vi "CFTS-Options Dialog.vi"(0 "Options in":T1, 2 "Parent VI":refnum<vi>) -> (4 "Options out":T1, 10 "Cancelled?":bool=TRUE)   [LabVIEW 2020]
doc: "Use this template to create a dialog box with event handling."
uses:
  epl-vi-lib/Utility VIs/Controls/KBackground Gradient/KBackground Gradient.xctl
  CFTS-Options.ctl
  epl-vi-lib/Utility VIs/Controls/KListboxEx/KListboxEx.xctl
panel:
  in  "Root data folder":path
  in  "Allow nonEPL":bool caption="Allow non-EPL compatible"
  in  "Names":i32(xcontrol)
  in  "Allow all users":bool
  in  "Users":i32(xcontrol)
  in  "Password":bool
  in  "Extension":string caption="Default data file extension"
  in  "Rig name":string
  in  "Help Button":bool
  in  "background":dbl(xcontrol)
  in  "Vitals":bool caption="Auto-start physiological monitor"
  in  "Left":u16(ring) items=["57TTH", "TTH66"]
  in  "Right":u16(ring) items=["57TTH", "TTH66"]
  in  "Cancel":bool
  in  "OK":bool
  # "Options"
  # "Acoustic System IDs"
  # "Other options"
  # "Advanced users"
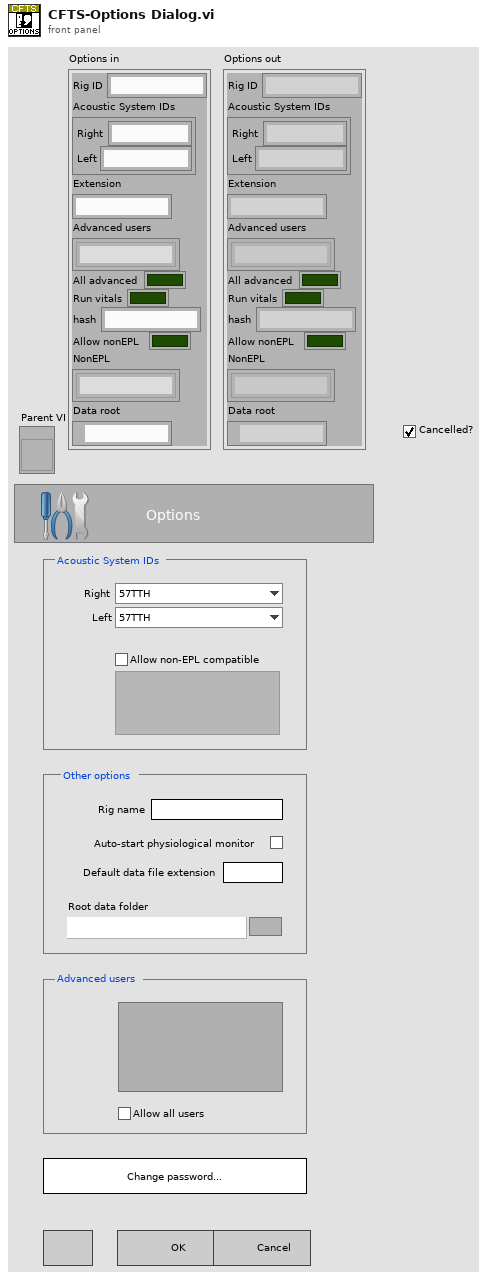
[diagram p1: front panel]
types:
  T1 = typedef "CFTS-Options.ctl" = cluster{"Rig ID":string, "Acoustic System IDs":cluster{"Right":string, "Left":string}, "Extension":string, "Advanced users":string[], "All advanced":bool, "Run vitals":bool, "hash":string, "Allow nonEPL":bool, "NonEPL":string[], "Data root":path}
  T2 = enum8{"Enabled", "Disabled", "Disabled and Grayed Out"}
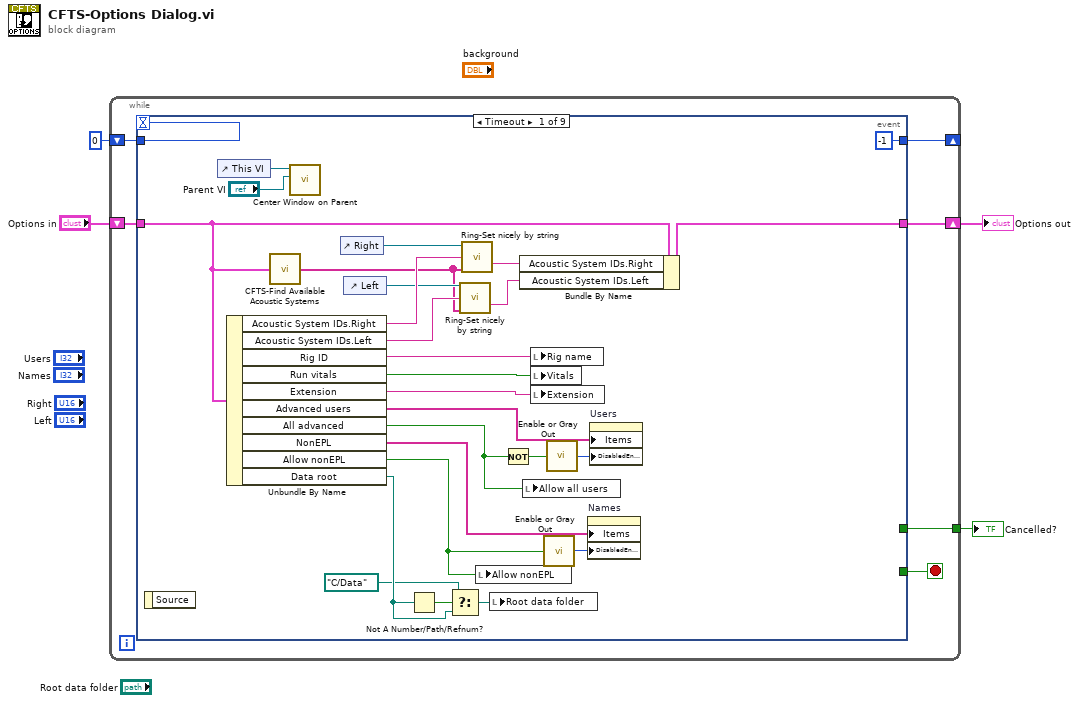
[diagram p0: block diagram]
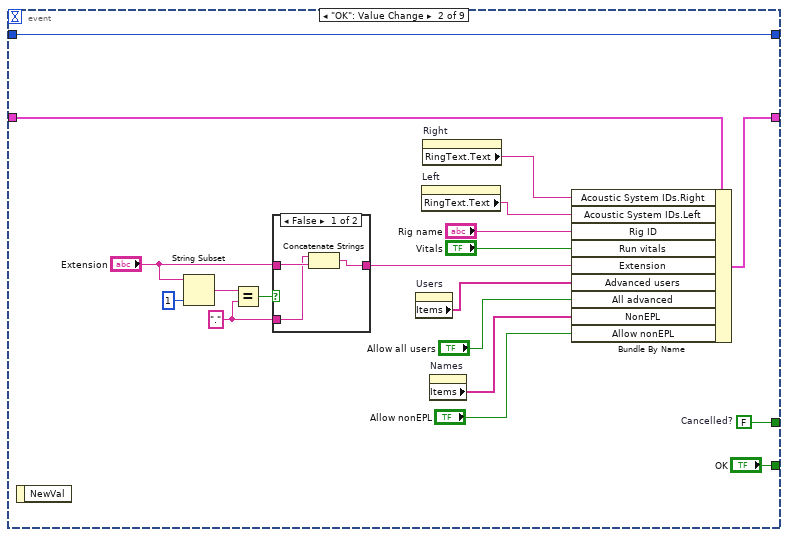
[diagram p2: hidden frame]
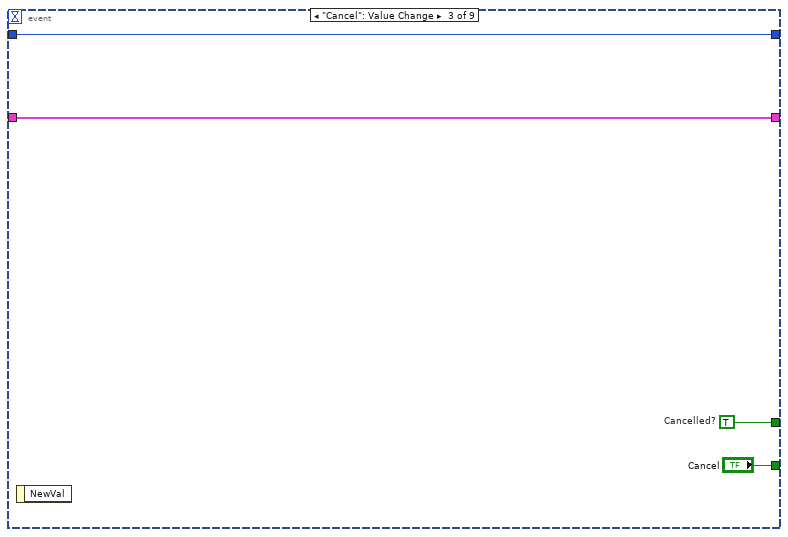
[diagram p4: hidden frame]
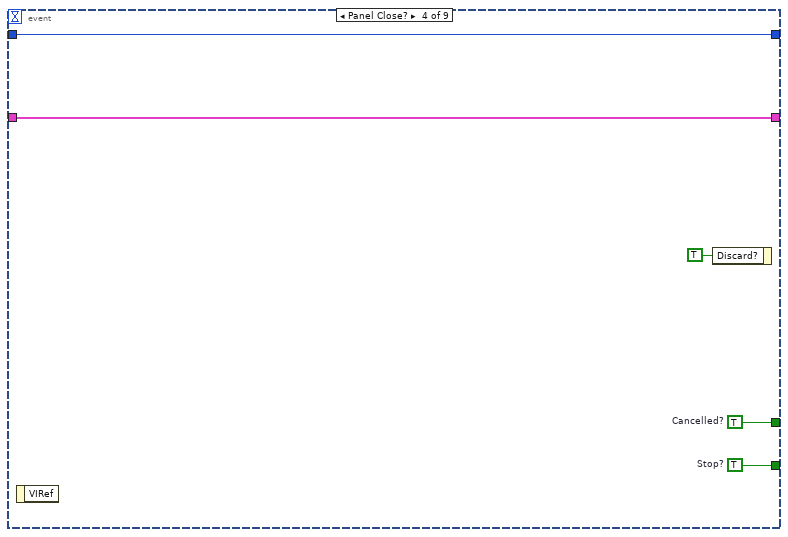
[diagram p5: hidden frame]
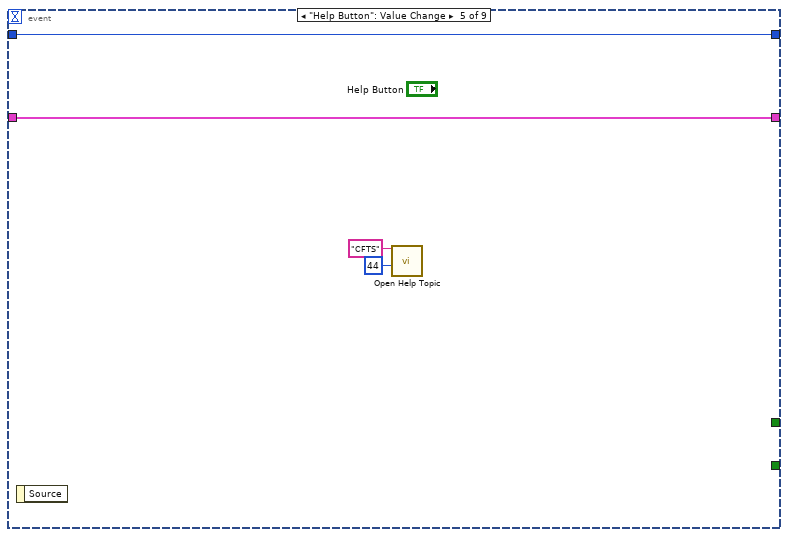
[diagram p6: hidden frame]
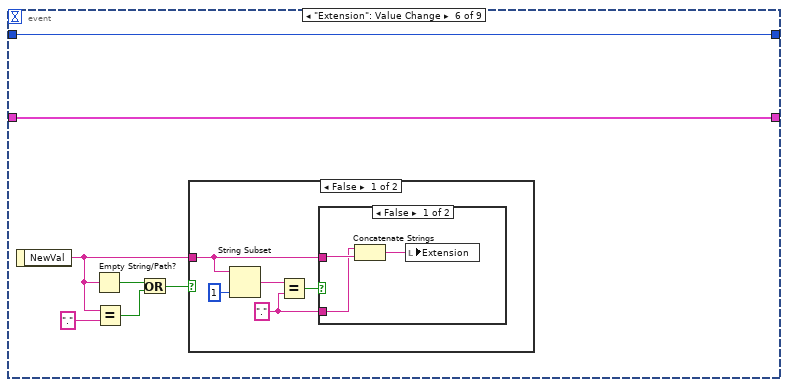
[diagram p7: hidden frame]
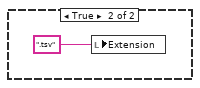
[diagram p9: hidden frame]
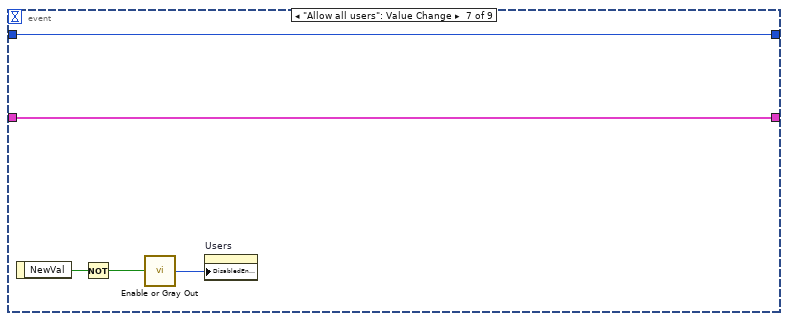
[diagram p10: hidden frame]
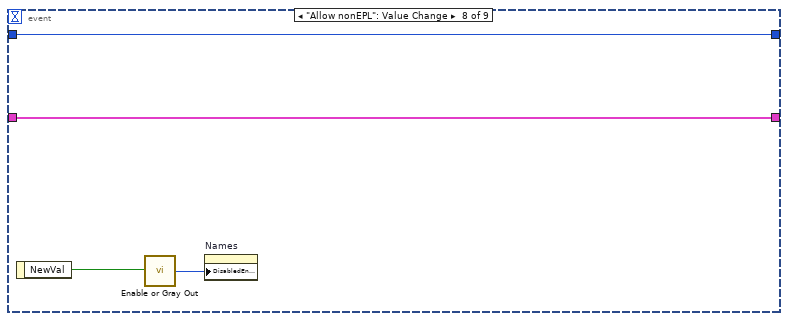
[diagram p11: hidden frame]
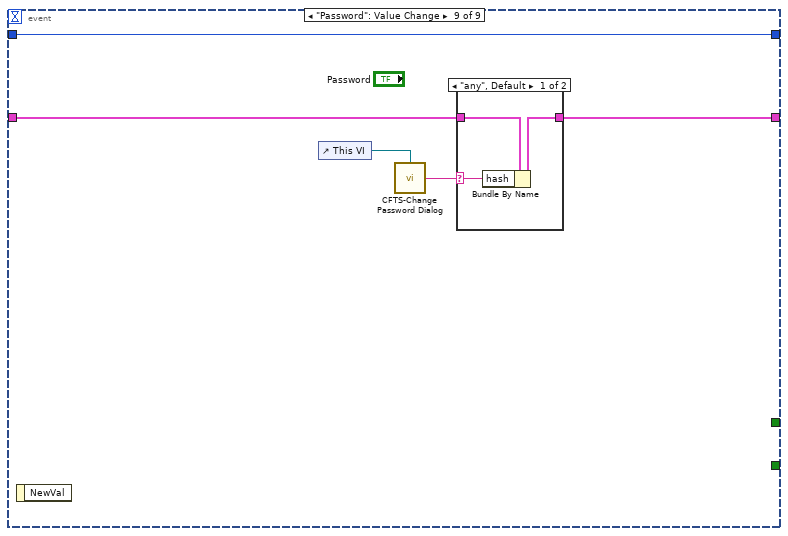
[diagram p12: hidden frame]
diagram:
  n1 = while {
    tunnel: [w9] -> w4
    shift-right: [w8] -> _
    shift-left: 0 -> [w7]
    shift-right: [w6] -> w1
    shift-left: "Options in" -> [w5]
    stop <- w10 stop-if-true
    n2 = event shown="[0] Timeout" {
      selector: _ -> [_ _ _ _ _ _ _ _ _]
      dyn-events: _ -> [_ _ _ _ _ _ _ _ _]
      timeout: w7 -> [_ _ _ _ _ _ _ _ _]
      tunnel: [_ "OK" "Cancel" w67 _ _ _ _ _] -> w10
      tunnel: [_ w55 w63 w66 _ _ _ _ _] -> w9
      tunnel: [-1 w52 w61 w65 w72 w79 w93 w97 w102] -> w8
      tunnel: w7 -> [_ w52 w61 w65 w72 w79 w93 w97 w102]
      tunnel: [w19 w45 w60 w64 w71 w78 w92 w96 w98] -> w6
      tunnel: w5 -> [w15 w51 w60 w64 w71 w78 w92 w96 w100]
      event Timeout {
        n3 = event-data() -> ()  [unwired: 1 in, 1 out]
        n4 = control-ref of="This VI"() -> (w32:refnum<vi>)
        n5 = Unbundle By Name(w15) -> ("Acoustic System IDs.Right"=w22:string, "Acoustic System IDs.Left"=w21:string, "Rig ID"=w33:string, "Run vitals"=w35:bool, "Extension"=w34:string, "Advanced users"=w30:string[], "All advanced"=w28:bool, "NonEPL"=w26:string[], "Allow nonEPL"=w24:bool, "Data root"=w12:path)
        n6 = call "CFTS-Find Available Acoustic Systems.vi"("Options"=w15) -> ("Acoustic Systems"=w16:string[])  [unwired: 14 in]
        n7 = call "Center Window on Parent.vi"("Parent VI"="Parent VI", "VI in"=w32) -> ()  [unwired: 8 in, 2 out]
        n8 = control-ref of="Right"() -> (w23:refnum<vi>)
        n9 = control-ref of="Left"() -> (w20:refnum<vi>)
        n10 = Not A Number/Path/Refnum?(number/path/refnum=w12) -> (NaN/Path/Refnum?=w14:bool)
        n11 = Select(t=path "C:/Data", s=w14, f=w12) -> (s? t:f=w13:path)
        n12 = call "Ring-Set nicely by string.vi"("Ring in"=w20, "Device"=w21, "Strings []"=w16) -> ("Selection"=w17:string)  [unwired: 8 in, 4 out]
        n13 = call "Ring-Set nicely by string.vi"("Ring in"=w23, "Device"=w22, "Strings []"=w16) -> ("Selection"=w18:string)  [unwired: 8 in, 4 out]
        n14 = local write "Allow nonEPL"(w24) -> ()
        n15 = local write "Root data folder"(w13) -> ()
        n16 = Not(x=w28) -> (.not. x?=w27:bool)
        n17 = Bundle By Name(cluster=w15, "Acoustic System IDs.Right"=w18, "Acoustic System IDs.Left"=w17) -> (w19:T1)
        n18 = local write "Allow all users"(w28) -> ()
        n19 = local write "Rig name"(w33) -> ()
        n20 = local write "Vitals"(w35) -> ()
        n21 = local write "Extension"(w34) -> ()
        n22 = call "Enable or Gray Out.vi"("Boolean"=w24) -> ("Disabled"=w25:T2)
        n23 = call "Enable or Gray Out.vi"("Boolean"=w27) -> ("Disabled"=w29:T2)
        n24 = property on="Names" class="KListboxEx (strict)"("Items"=w26, "DisabledEnum"=w25) -> ()  [unwired: 2 in, 2 out]
        n25 = property on="Users" class="KListboxEx (strict)"("Items"=w30, "DisabledEnum"=w29) -> ()  [unwired: 2 in, 2 out]
      }
      event "OK": Value Change {
        w46 = "."
        w55 = FALSE  # Cancelled?
        n26 = event-data() -> ()  [unwired: 1 in, 1 out]
        n27 = String Subset(string="Extension", length (rest)=1 ("length (rest)")) -> (substring=w49:string)  [unwired: 1 in]
        n28 = Equal?(x=w49, y=w46) -> (x = y?=w48:bool)
        n29 = case shown="False" w48 {
          tunnel: "Extension" -> [w58 w59]
          tunnel: w46 -> [w57 _]
          tunnel: [w56 w59] -> w43
          frame False {
            n30 = Concatenate Strings(w57, w58) -> (w56:string)
          }
          frame True {
          }
        }
        n31 = property on="Users" class="KListboxEx (strict)"() -> ("Items"=w42:string[])  [unwired: 2 in, 2 out]
        n32 = property on="Left" class="Ring (strict)"() -> ("RingText.Text"=w37:string)  [unwired: 2 in, 2 out]
        n33 = property on="Right" class="Ring (strict)"() -> ("RingText.Text"=w38:string)  [unwired: 2 in, 2 out]
        n34 = property on="Names" class="KListboxEx (strict)"() -> ("Items"=w40:string[])  [unwired: 2 in, 2 out]
        n35 = Bundle By Name(cluster=w51, "Acoustic System IDs.Right"=w38, "Acoustic System IDs.Left"=w37, "Rig ID"="Rig name", "Run vitals"="Vitals", "Extension"=w43, "Advanced users"=w42, "All advanced"="Allow all users", "NonEPL"=w40, "Allow nonEPL"="Allow nonEPL") -> (w45:T1)
      }
      event "Cancel": Value Change {
        w63 = TRUE  # Cancelled?
        n36 = event-data() -> ()  [unwired: 1 in, 1 out]
      }
      event Panel Close? {
        w66 = TRUE  # Cancelled?
        w67 = TRUE  # Stop?
        n37 = event-data() -> ()  [unwired: 1 in, 1 out]
        n38 = event-data("Discard?"=TRUE) -> ()  [unwired: 1 in, 1 out]
      }
      event "Help Button": Value Change {
        n39 = event-data() -> ()  [unwired: 1 in, 1 out]
        n40 = call "Open Help Topic.vi"("Help file"="CFTS", "HelpId"=44) -> ()  [unwired: 13 in, 1 out]
      }
      event "Extension": Value Change {
        n41 = event-data() -> ("NewVal"=w76:string)  [unwired: 1 in]
        n42 = Empty String/Path?(string/path=w76) -> (empty?=w77:bool)
        n43 = Equal?(x=w76, y=".") -> (x = y?=w73:bool)
        n44 = Or(x=w77, y=w73) -> (x .or. y?=w74:bool)
        n45 = case shown="False" w74 {
          tunnel: w76 -> [w80 _]
          frame False {
            w82 = "."
            n46 = String Subset(string=w80, length (rest)=1 ("length (rest)")) -> (substring=w83:string)  [unwired: 1 in]
            n47 = Equal?(x=w83, y=w82) -> (x = y?=w81:bool)
            n48 = case shown="False" w81 {
              tunnel: w80 -> [w87 _]
              tunnel: w82 -> [w86 _]
              frame False {
                n49 = Concatenate Strings(w86, w87) -> (w85:string)
                n50 = local write "Extension"(w85) -> ()
              }
              frame True {
              }
            }
          }
          frame True {
            n51 = local write "Extension"(".tsv") -> ()
          }
        }
      }
      event "Allow all users": Value Change {
        n52 = event-data() -> ("NewVal"=w91:bool)  [unwired: 1 in]
        n53 = Not(x=w91) -> (.not. x?=w89:bool)
        n54 = call "Enable or Gray Out.vi"("Boolean"=w89) -> ("Disabled"=w90:T2)
        n55 = property on="Users" class="KListboxEx (strict)"("DisabledEnum"=w90) -> ()  [unwired: 2 in, 2 out]
      }
      event "Allow nonEPL": Value Change {
        n56 = event-data() -> ("NewVal"=w94:bool)  [unwired: 1 in]
        n57 = call "Enable or Gray Out.vi"("Boolean"=w94) -> ("Disabled"=w95:T2)
        n58 = property on="Names" class="KListboxEx (strict)"("DisabledEnum"=w95) -> ()  [unwired: 2 in, 2 out]
      }
      event "Password": Value Change {
        n59 = event-data() -> ()  [unwired: 1 in, 1 out]
        n60 = control-ref of="This VI"() -> (w101:refnum<vi>)
        n61 = call "CFTS-Change Password Dialog.vi"("Parent VI"=w101) -> ("hash"=w99:string)  [unwired: 14 in]
        n62 = case shown="\"any\", Default" w99 {
          selector: w99 -> [w103 _]
          tunnel: w100 -> [w105 w106]
          tunnel: [w104 w106] -> w98
          frame "any", Default {
            n63 = Bundle By Name(cluster=w105, "hash"=w103) -> (w104:T1)
          }
          frame "" {
          }
        }
      }
    }
  }
  "Cancelled?" <- w4
  "Options out" <- w1
